vi "Close Hardware References.vi"(8 "error in (no error)":errorcluster, 11 "HW Refnum in":string) -> (0 "error out":errorcluster, 3 "HW Refnum out":string)   [LabVIEW 2018, in "LGP5 Acquisition.lvlib" / "DAQ Device.lvlib"]
doc: "Close the hardware references.\n_____\nBased on Delacor QMH Project Template 4.2.0.62."
uses:
  DAQ Device.lvlib
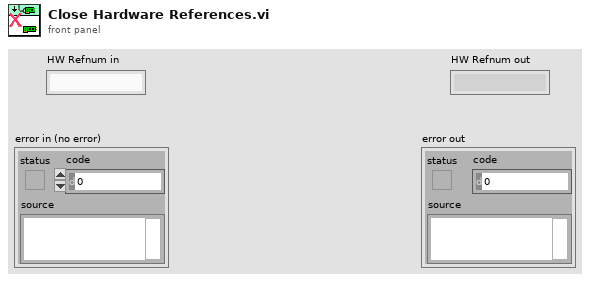
[diagram p1: front panel]
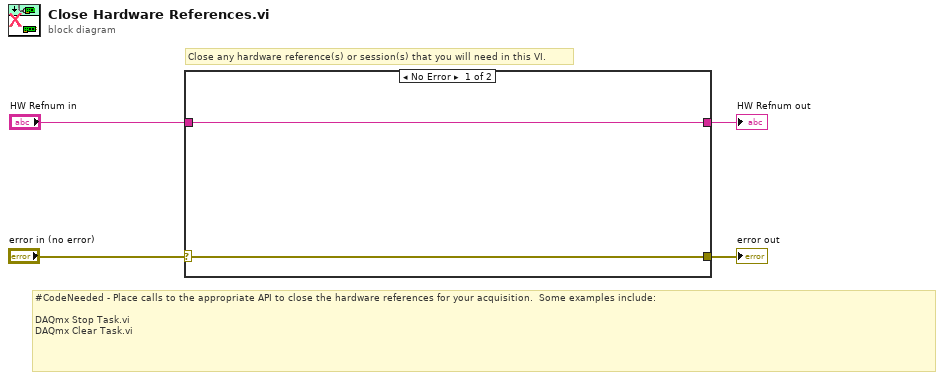
[diagram p0: block diagram]
diagram:
  # "Close any hardware reference(s) or session(s) that you will need in this VI."
  # "#CodeNeeded - Place calls to the appropriate API to close the hardware references for your acquisition.  Some examples include:\n\nDAQmx Stop Task.vi\nDAQmx Clear Task.vi"
  n1 = case shown="No Error" "error in (no error)" {
    selector: "error in (no error)" -> [w6 w7]
    tunnel: [w6 w7] -> w3
    tunnel: "HW Refnum in" -> [w5 w8]
    tunnel: [w5 w8] -> w1
    frame No Error {
    }
    frame Error {
    }
  }
  "HW Refnum out" <- w1
  "error out" <- w3
